vi "FileLogTargetCtl.vi"(6 "Actual Start [f] in":i64, 7 "Actual Start [f] 3":i64, 8 "error in (no error)":errorcluster, 9 "Log-Target":bool, 10 "Output - Cluster":T1 {"TS-5 [°C]" format="%#.2g"; "pHS-1 [pH]" format="%.2g"; "TS-4 [°C]" format="%#.2g"; "FS-2 [l]" format="%.2g"; "FS-1 [l]" format="%.2g"; "DS-1 [bar]" format="%#.2g"; "DFS-1 [l/min]" format="%#.2g"; "FS-3 [l]" format="%.2g"; "DFS-1 [dl]" format="%.0g"}, 11 "Byte Stream File in":refnum<file>) -> (0 "error out":errorcluster, 2 "Actual Start [f] out":i64, 3 "Byte Stream File out":refnum<file>)   [LabVIEW 2011]
uses:
  Output - Cluster b2g2.ctl
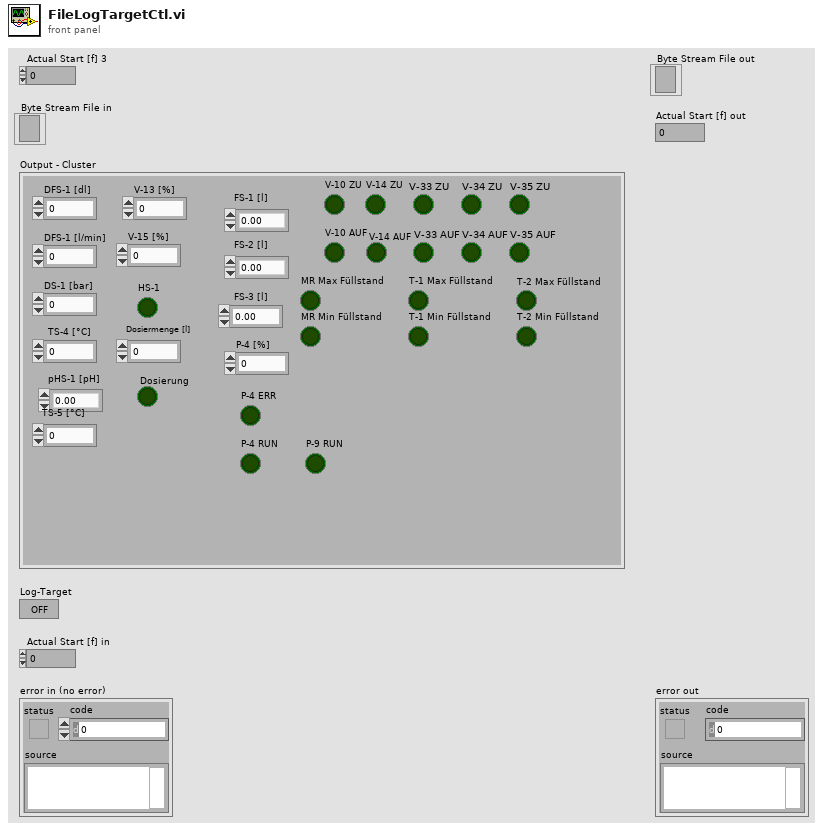
[diagram p1: front panel]
types:
  T1 = typedef "Output - Cluster b2g2.ctl" = cluster{"DFS-1 [dl]":u64, "FS-3 [l]":dbl, "DFS-1 [l/min]":dbl, "DS-1 [bar]":dbl, "V-10 ZU":bool, "V-14 ZU":bool, "FS-1 [l]":dbl, "FS-2 [l]":dbl, "TS-4 [°C]":dbl, "HS-1":bool, "V-13 [%]":u8, "V-15 [%]":u8, "P-4 [%]":u8, "Dosierung":bool, "MR Max Füllstand":bool, "MR Min Füllstand":bool, "Dosiermenge [l]":sgl, "V-14 AUF":bool, "V-10 AUF":bool, "T-1 Max Füllstand":bool, "T-1 Min Füllstand":bool, "T-2 Max Füllstand":bool, "T-2 Min Füllstand":bool, "pHS-1 [pH]":dbl, "P-4 RUN":bool, "V-33 AUF":bool, "V-33 ZU":bool, "V-34 AUF":bool, "V-34 ZU":bool, "P-4 ERR":bool, "TS-5 [°C]":dbl, "V-35 AUF":bool, "V-35 ZU":bool, "P-9 RUN":bool}
  T2 = enum16{"open", "replace", "create", "open or create", "replace or create", "replace or create with confirmation"}
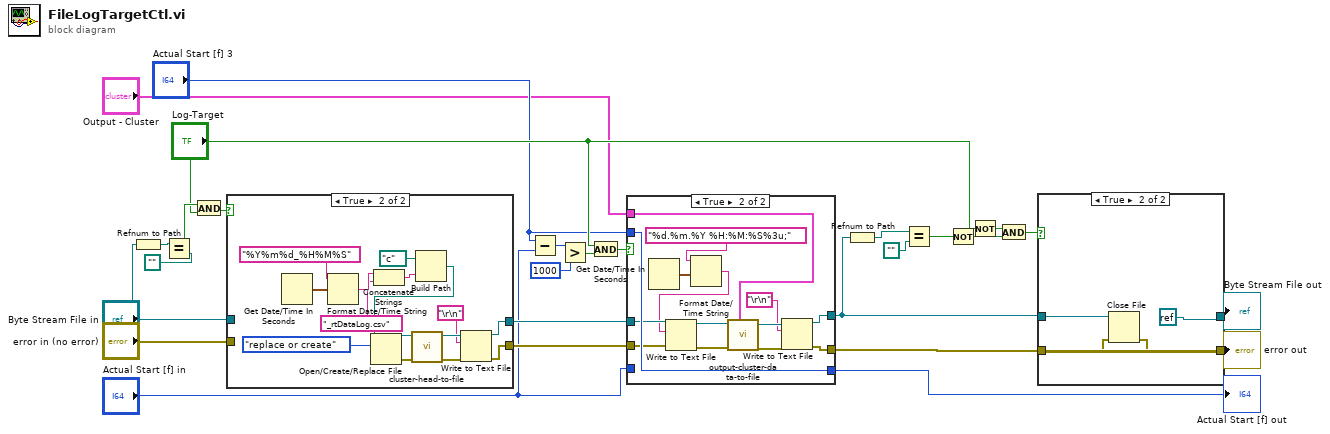
[diagram p0: block diagram]
diagram:
  n1 = Refnum to Path(1:"Byte Stream File in") -> (0:w22:path)
  n2 = Equal?(x=w22, y=path "") -> (x = y?=w26:bool)
  n3 = And(x=w26, y="Log-Target") -> (x .and. y?=w25:bool)
  n4 = case shown="True" w25 {
    tunnel: [w29 w31] -> w20
    tunnel: [w28 w32] -> w21
    tunnel: "Byte Stream File in" -> [w29 _]
    tunnel: "error in (no error)" -> [w28 _]
    frame False {
    }
    frame True {
      n5 = Get Date/Time In Seconds() -> (seconds since 1Jan1904=w42:timestamp)
      n6 = Format Date/Time String(time format string (%c)="%Y%m%d_%H%M%S", seconds (now)=w42) -> (date/time string=w41:string)  [unwired: 1 in]
      n7 = Concatenate Strings(w41, "_rtDataLog.csv" ("name or relative path")) -> (w38:string)
      n8 = Build Path(base path=path "c:/", name or relative path=w38) -> (appended path=w37:path)
      n9 = Open/Create/Replace File(file path (use dialog)=w37, operation (0:open)=T2."replace or create") -> (refnum out=w36:refnum<file>, error out=w35:errorcluster)  [unwired: 4 in, 1 out]
      n10 = call "cluster-head-to-file.vi"("refnum in"=w36, "error in"=w35) -> ("refnum out"=w34:refnum<file>, "error out"=w33:errorcluster)  [unwired: 7 in]
      n11 = Write to Text File(file (use dialog)=w34, text="\r\n", error in=w33) -> (refnum out=w31:refnum<file>, error out=w32:errorcluster)  [unwired: 1 in, 1 out]
    }
  }
  n12 = Subtract(x="Actual Start [f] 3", y="Actual Start [f] in") -> (x-y=w2:i64)
  n13 = Greater?(x=w2, y=i64 1000) -> (0:w4:bool)
  n14 = And(x="Log-Target", y=w4) -> (x .and. y?=w5:bool)
  n15 = case shown="True" w5 {
    tunnel: [w45 w56] -> w12
    tunnel: [w46 w57] -> w10
    tunnel: "Output - Cluster" -> [_ w61]
    tunnel: "Actual Start [f] 3" -> [_ w60]
    tunnel: [w47 w60] -> w18
    tunnel: "Actual Start [f] in" -> [w47 _]
    tunnel: w20 -> [w45 w54]
    tunnel: w21 -> [w46 w53]
    frame False {
    }
    frame True {
      n16 = Get Date/Time In Seconds() -> (seconds since 1Jan1904=w49:timestamp)
      n17 = Format Date/Time String(time format string (%c)="%d.%m.%Y %H:%M:%S%3u;", seconds (now)=w49) -> (date/time string=w48:string)  [unwired: 1 in]
      n18 = Write to Text File(file (use dialog)=w54, text=w48, error in=w53) -> (refnum out=w51:refnum<file>, error out=w52:errorcluster)  [unwired: 1 in, 1 out]
      n19 = call "output-cluster-data-to-file.vi"("refnum in"=w51, "error in"=w52, "Output - Cluster"=w61) -> ("refnum out"=w59:refnum<file>, "error out"=w58:errorcluster)  [unwired: 6 in]
      n20 = Write to Text File(file (use dialog)=w59, text="\r\n", error in=w58) -> (refnum out=w56:refnum<file>, error out=w57:errorcluster)  [unwired: 1 in, 1 out]
    }
  }
  "Actual Start [f] out" <- w18
  n21 = Refnum to Path(1:w12) -> (0:w13:path)
  n22 = Equal?(x=w13, y=path "") -> (x = y?=w15:bool)
  n23 = Not(x=w15) -> (.not. x?=w17:bool)
  n24 = Not(x="Log-Target") -> (.not. x?=w16:bool)
  n25 = And(x=w16, y=w17) -> (x .and. y?=w11:bool)
  n26 = case shown="True" w11 {
    tunnel: [w63 refnum<k0> refnum] -> w8
    tunnel: w12 -> [w63 w67]
    tunnel: [w62 w65] -> w9
    tunnel: w10 -> [w62 w66]
    frame False {
    }
    frame True {
      n27 = Close File(refnum=w67, error in=w66) -> (error out=w65:errorcluster)  [unwired: 1 out]
    }
  }
  "error out" <- w9
  "Byte Stream File out" <- w8
